vi "getMFC_ring2.vi"() -> ()   [LabVIEW 2011]
uses:
  MFC_ring.ctl
  globals.vi
panel:
  out "output array":string[](array[string])
  in  "Tab Control":enum32{"Page 1", "Page 2"}(tab)
  in  "D/A Cards":T2 {"D/A (12-bit) Card"."Channel"."Channel" items=["N2 flow (NMFC1)", "H2 flow (HMFC1)", "Al flow (AlMFC1)"]; "Quad D/A (10-bit) Cards"."Channels 4"."Channel 4" items=["flow 1", "flow 2", "flow 3"]; "Quad D/A (10-bit) Cards"."Channels 4"."Channel 3" items=["flow 1", "flow 2", "flow 3"]; "Quad D/A (10-bit) Cards"."Channels 4"."Channel 2" items=["flow 1", "flow 2", "flow 3"]; "Quad D/A (10-bit) Cards"."Channels 4"."Channel 1" items=["flow 1", "flow 2", "flow 3"]; "Quad D/A (10-bit) Cards"."Channels 3"."Channel 4" items=["flow 1", "flow 2", "flow 3"]; "Quad D/A (10-bit) Cards"."Channels 3"."Channel 3" items=["flow 1", "flow 2", "flow 3"]; "Quad D/A (10-bit) Cards"."Channels 3"."Channel 2" items=["flow 1", "flow 2", "flow 3"]; "Quad D/A (10-bit) Cards"."Channels 3"."Channel 1" items=["flow 1", "flow 2", "flow 3"]; "Quad D/A (10-bit) Cards"."Channels 2"."Channel 4" items=["flow 1", "flow 2", "flow 3"]; "Quad D/A (10-bit) Cards"."Channels 2"."Channel 3" items=["flow 1", "flow 2", "flow 3"]; "Quad D/A (10-bit) Cards"."Channels 2"."Channel 2" items=["flow 1", "flow 2", "flow 3"]; "Quad D/A (10-bit) Cards"."Channels 2"."Channel 1" items=["flow 1", "flow 2", "flow 3"]; "Quad D/A (10-bit) Cards"."Channels"."Channel 4" items=["flow 1", "flow 2", "flow 3"]; "Quad D/A (10-bit) Cards"."Channels"."Channel 3" items=["flow 1", "flow 2", "flow 3"]; "Quad D/A (10-bit) Cards"."Channels"."Channel 2" items=["flow 1", "flow 2", "flow 3"]; "Quad D/A (10-bit) Cards"."Channels"."Channel 1" items=["flow 1", "flow 2", "flow 3"]; "Quad D/A (10-bit) Cards"."Channels"."Channel 4" items=["flow 1", "flow 2", "flow 3"]; "Quad D/A (10-bit) Cards"."Channels"."Channel 3" items=["flow 1", "flow 2", "flow 3"]; "Quad D/A (10-bit) Cards"."Channels"."Channel 2" items=["flow 1", "flow 2", "flow 3"]; "Quad D/A (10-bit) Cards"."Channels"."Channel 1" items=["N2 flow (NMFC1)", "H2 flow (HMFC1)", "Al flow (ALMFC1)", "Ga flow 1 (GAMFC1)", "Ga flow 2 (GAMFC2)", "Ga flow 3 (GAMFC3)", "In flow (INMFC1)"]}
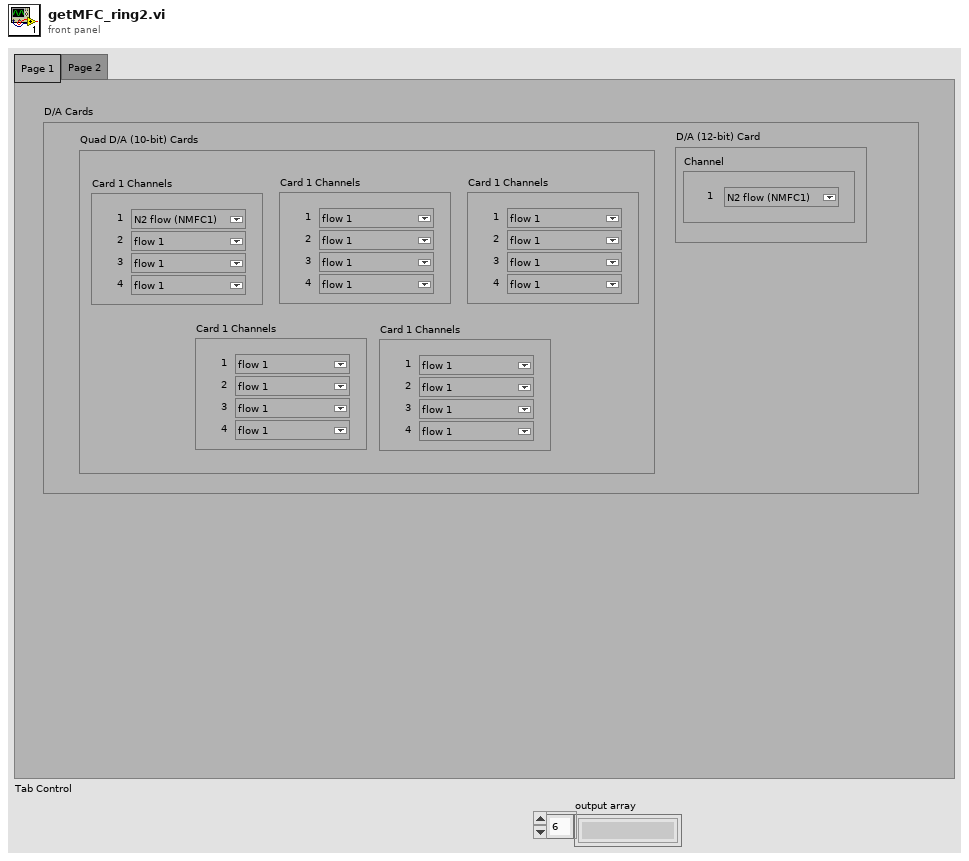
[diagram p1: front panel]
types:
  T1 = typedef "MFC_ring.ctl" = u16
  T2 = cluster{"Quad D/A (10-bit) Cards":cluster{"Channels":cluster{"Channel 1":u16, "Channel 2":u16, "Channel 3":u16, "Channel 4":u16}, "Channels":cluster{"Channel 1":u16, "Channel 2":u16, "Channel 3":u16, "Channel 4":u16}, "Channels 2":cluster{"Channel 1":u16, "Channel 2":u16, "Channel 3":u16, "Channel 4":u16}, "Channels 3":cluster{"Channel 1":u16, "Channel 2":u16, "Channel 3":u16, "Channel 4":u16}, "Channels 4":cluster{"Channel 1":u16, "Channel 2":u16, "Channel 3":u16, "Channel 4":u16}}, "D/A (12-bit) Card":cluster{"Channel":cluster{"Channel":T1}}}
  T3 = cluster{"NMFC1":cluster{"MFC Range":u16, "MFC Name":string}, "HMFC1":cluster{"MFC Range":u16, "MFC Name":string}, "ALMFC1":cluster{"MFC Range":u16, "MFC Name":string}, "ALMFC1 2":cluster{"MFC Range":u16, "MFC Name":string}, "ALMFC1 3":cluster{"MFC Range":u16, "MFC Name":string}, "ALMFC1 4":cluster{"MFC Range":u16, "MFC Name":string}, "ALMFC1 5":cluster{"MFC Range":u16, "MFC Name":string}}
  T4 = cluster{"Channels":cluster{"Channel 1":u16, "Channel 2":u16, "Channel 3":u16, "Channel 4":u16}, "Channels":cluster{"Channel 1":u16, "Channel 2":u16, "Channel 3":u16, "Channel 4":u16}, "Channels 2":cluster{"Channel 1":u16, "Channel 2":u16, "Channel 3":u16, "Channel 4":u16}, "Channels 3":cluster{"Channel 1":u16, "Channel 2":u16, "Channel 3":u16, "Channel 4":u16}, "Channels 4":cluster{"Channel 1":u16, "Channel 2":u16, "Channel 3":u16, "Channel 4":u16}}
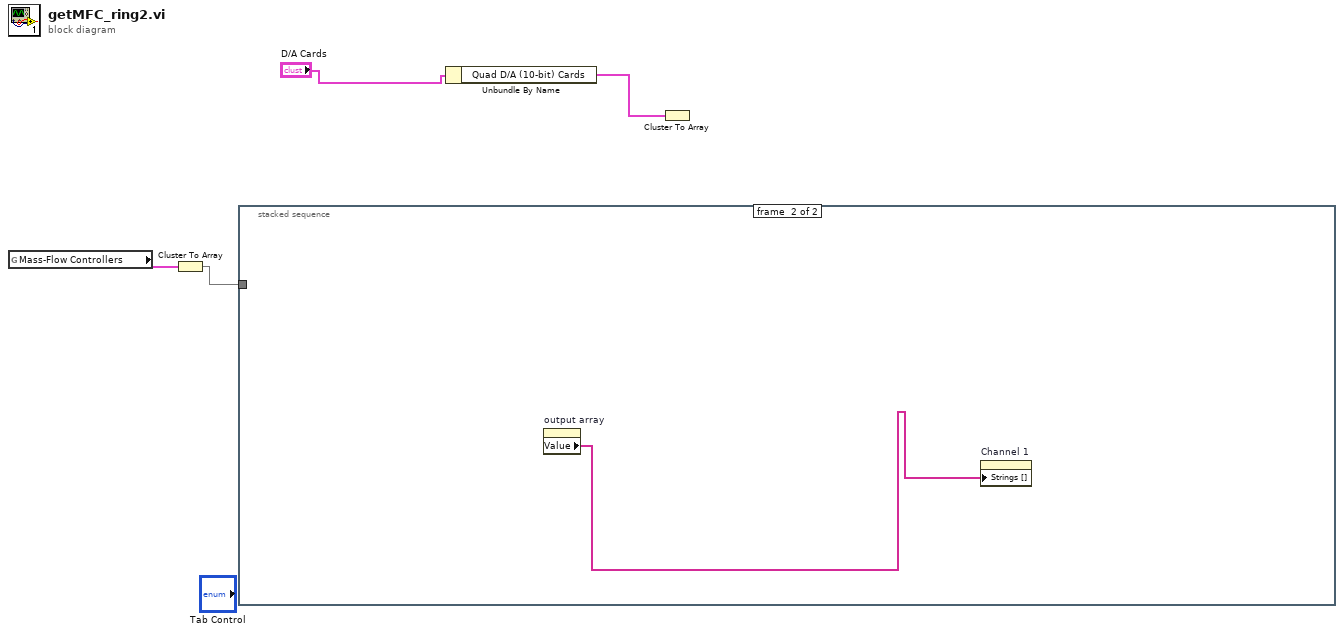
[diagram p0: block diagram]
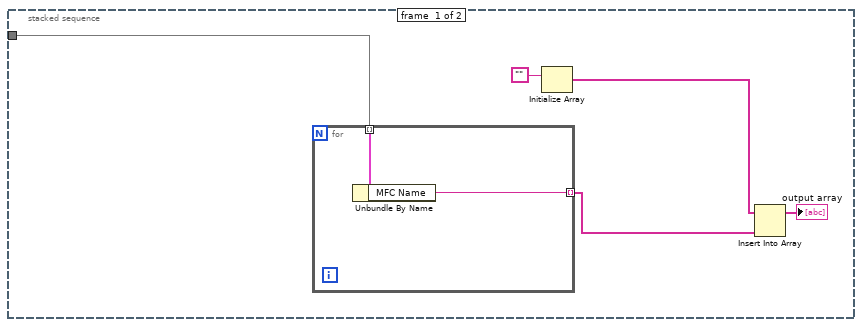
[diagram p2: hidden frame]
diagram:
  n1 = global read "globals.vi" "Mass-Flow Controllers"() -> (w4:T3)
  n2 = Cluster To Array(cluster=w4) -> (array=w3:cluster{"MFC Range":u16, "MFC Name":string}[])
  n3 = stacked-sequence {
    tunnel: w3 -> [w6 _]
    frame #0 {
      n4 = for {
        tunnel: w6 -> [w11] mode=indexing
        tunnel: [w10] -> w8 mode=indexing
        n5 = Unbundle By Name(w11) -> ("MFC Name"=w10:string)
      }
      n6 = Initialize Array("") -> (w7:string[])  [unwired: 1 in]
      n7 = Insert Into Array(array=w7, new element=w8) -> (→"output array":string[])  [unwired: 1 in]
    }
    frame #1 {
      n8 = property on="output array" class="Arr (strict)"() -> ("Value"=w12:string[])  [unwired: 2 in, 2 out]
      n9 = property on="Channel 1" class="Ring (strict)"("Strings []"=w12) -> ()  [unwired: 2 in, 2 out]
    }
  }
  n10 = Unbundle By Name("D/A Cards") -> ("Quad D/A (10-bit) Cards"=w2:T4)
  n11 = Cluster To Array(cluster=w2) -> ()  [unwired: 1 out]
